vi "get_config_cluster.vi"(8 "error in (no error)":errorcluster, 11 "FPGAWrapperDL090211Galvo in":refnum<class "FPGAWrapperDL090211Galvo_grabber.lvclass">) -> (0 "error out":errorcluster, 2 "config cluster (variant)":variant, 3 "FPGAWrapperDL090211Galvo out":refnum<class "FPGAWrapperDL090211Galvo_grabber.lvclass">)   [LabVIEW 2010, in "FPGAWrapperDL090211Galvo_grabber.lvclass"]
uses:
  FPGAWrapperDL090211Galvo_grabber.lvclass
  FPGAWrapperDL090211Galvo_grabber.lvclass/FPGAWrapperDL090211Galvo_grabber.ctl
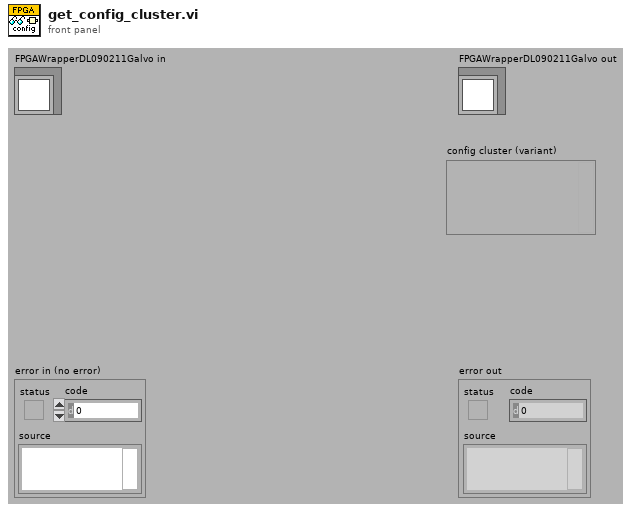
[diagram p1: front panel]
types:
  T1 = typedef "config_data_cluster.ctl" = cluster{"bit file":string, "hifo box version":i32, "ADC clock phase":i32}
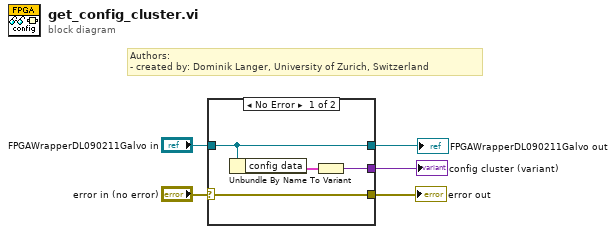
[diagram p0: block diagram]
diagram:
  # "Authors: \n- created by: Dominik Langer, University of Zurich, Switzerland"
  n1 = case shown="No Error" "error in (no error)" {
    selector: "error in (no error)" -> [w6 w11]
    tunnel: "FPGAWrapperDL090211Galvo in" -> [w9 w10]
    tunnel: [w7 _] -> w3
    tunnel: [w6 w11] -> w2
    tunnel: [w9 w10] -> w1
    frame No Error {
      n2 = Unbundle By Name(w9) -> ("config data"=w8:T1)
      n3 = To Variant(anything=w8) -> (Variant=w7:variant)
    }
    frame Error {
    }
  }
  "error out" <- w2
  "FPGAWrapperDL090211Galvo out" <- w1
  "config cluster (variant)" <- w3
